vi "Fluke8808_Config.vi"(0 "MyIndex":u8, 1 "Measurement Function":u16(ring) items=["DC Volts", "AC Volts", "DC Current", "AC Current", "2-Wire Resistance", "4-Wire Resistance", "Frequency", "AC and DC rms Current", "AC and DC rms Volts", "Continuity", "Diode"], 2 "Measurement Rate":u16(ring)=1 items=["Slow", "Medium", "Fast"], 3 "Decibel Reference Impedance":u16(ring)=1 items=["2 Ohms"=1, "4 Ohms"=2, "8 Ohms"=3, "16 Ohms"=4, "50 Ohms"=5, "75 Ohms"=6, "93 Ohms"=7, "110 Ohms"=8, "124 Ohms"=9, "125 Ohms"=10, "135 Ohms"=11, "150 Ohms"=12, "250 Ohms"=13, "300 Ohms"=14, "500 Ohms"=15, "600 Ohms"=16, "800 Ohms"=17, "900 Ohms"=18, "1000 Ohms"=19, "1200 Ohms"=20, "8000 Ohms"=21], 5 "Measurement Modifier":u16(ring) items=["None", "Decibels", "Decibel Power"], 7 "Enable Range":bool=TRUE, 9 "Manual Range":u16(ring)=5 items=["200 mV, 200 Ohms, 20 mA AC, 2 kHz, 200 miuA DC"=1, " 2 V, 2 kOhms, 200 mA AC, 20 kHz, 2000 miuA DC"=2, "20 V, 20 kOhms, 2 A AC, 200 kHz, 20 mA DC"=3, "200 V, 200 kOhms, 10 A AC, 1000 kHz, 200 mA DC"=4, "1000 V DC, 2 MOhms, 2 A DC"=5, "20 MOhms, 10 A DC"=6, "100 MOhms"=7], 11 "error in":errorcluster) -> (4 "OK?":bool, 15 "error out":errorcluster)   [LabVIEW 2015]
doc: "Configures the measurement type, resolution, and range on the instrument."
panel:
  in  "等待时间（毫秒）":u32
  out "VISA resource name out":refnum<visa-resource-name>
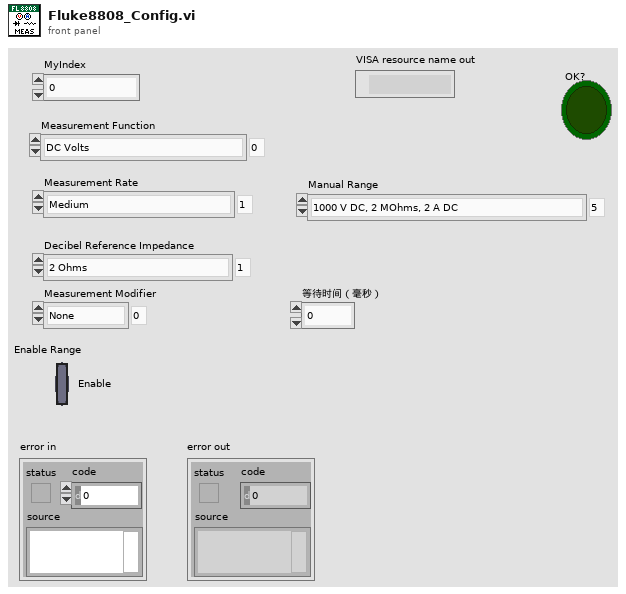
[diagram p1: front panel]
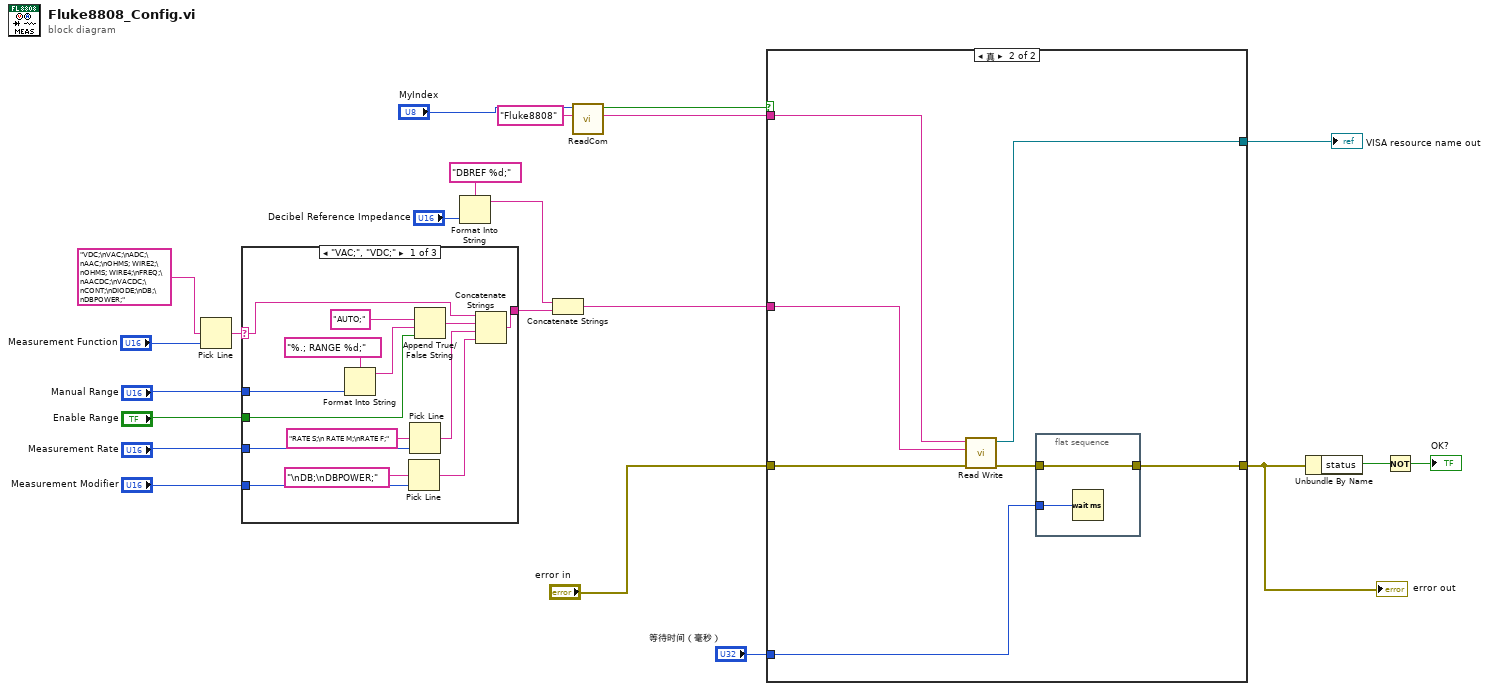
[diagram p0: block diagram]
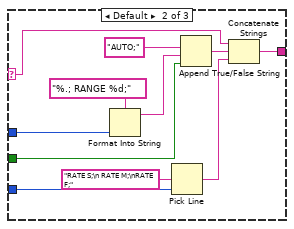
[diagram p3: hidden frame]
diagram:
  n1 = Pick Line(multi-line string="VDC;\nVAC;\nADC;\nAAC;\nOHMS; WIRE2;\nOHMS; WIRE4;\nFREQ;\nAACDC;\nVACDC;\nCONT;\nDIODE;\nDB;\nDBPOWER;" ("Measurement Function"), line index="Measurement Function") -> (output string=w20:string)  [unwired: 1 in]
  n2 = case shown="\"VAC;\", \"VDC;\"" w20 {
    selector: w20 -> [w23 w37 w48]
    tunnel: "Manual Range" -> [w27 w41 _]
    tunnel: "Enable Range" -> [w26 w40 _]
    tunnel: [w28 w38 w48] -> w17
    tunnel: "Measurement Rate" -> [w25 w39 _]
    tunnel: "Measurement Modifier" -> [w24 _ _]
    frame "VAC;", "VDC;" {
      n3 = Format Into String(format string="%.; RANGE %d;" ("Manual Range"), w27) -> (resulting string=w35:string)  [unwired: 2 in, 1 out]
      n4 = Pick Line(multi-line string="\nDB;\nDBPOWER;" ("Decibel and Db Power"), line index=w24) -> (output string=w29:string)  [unwired: 1 in]
      n5 = Pick Line(multi-line string="RATE S;\n RATE M;\nRATE F;" ("Measurement Rate"), line index=w25) -> (output string=w33:string)  [unwired: 1 in]
      n6 = Append True/False String(1:w26, 2:w35, 3:"AUTO;" ("Auto Range")) -> (0:w31:string)  [unwired: 1 in]
      n7 = Concatenate Strings(w23, w31, w33, w29) -> (w28:string)
    }
    frame Default {
      n8 = Format Into String(format string="%.; RANGE %d;" ("Manual Range"), w41) -> (resulting string=w46:string)  [unwired: 2 in, 1 out]
      n9 = Pick Line(multi-line string="RATE S;\n RATE M;\nRATE F;" ("Measurement Rate"), line index=w39) -> (output string=w44:string)  [unwired: 1 in]
      n10 = Append True/False String(1:w40, 2:w46, 3:"AUTO;" ("Auto Range")) -> (0:w42:string)  [unwired: 1 in]
      n11 = Concatenate Strings(w37, w42, w44) -> (w38:string)
    }
    frame "CONT;", "DIODE;" {
    }
  }
  n12 = Format Into String(format string="DBREF %d;" ("Decibel Reference Impedance"), "Decibel Reference Impedance") -> (resulting string=w18:string)  [unwired: 2 in, 1 out]
  n13 = Concatenate Strings(w18, w17) -> (w16:string)
  n14 = call "ReadCom.vi"("仪器名称"="Fluke8808", "MyIndex"="MyIndex") -> ("COM"=w6:string, "OK?"=w4:bool)  [unwired: 7 in, 1 out]
  n15 = case shown="真" w4 {
    tunnel: "error in" -> [w49 w56]
    tunnel: w16 -> [_ w55]
    tunnel: [_ w54] -> w9
    tunnel: w6 -> [_ w53]
    tunnel: [w49 w51] -> w3
    tunnel: "等待时间（毫秒）" -> [_ w50]
    frame False {
    }
    frame True {
      n16 = call "Read Write.vi"("error in (no error)"=w56, "Write String"=w55, "VISA resource name"=w53) -> ("error out"=w52:errorcluster, "VISA resource name out"=w54:refnum<visa-resource-name>)  [unwired: 6 in, 1 out]
      n17 = flat-sequence {
        tunnel: w52 -> [w58]
        tunnel: [w58] -> w51
        tunnel: w50 -> [w57]
        frame #0 {
          n18 = Wait (ms)(milliseconds to wait=w57) -> ()  [unwired: 1 out]
        }
      }
    }
  }
  "error out" <- w3
  "VISA resource name out" <- w9
  n19 = Unbundle By Name(w3) -> ("status"=w2:bool)
  n20 = Not(x=w2) -> (.not. x?=→"OK?":bool)
